vi "UHR-Fleezers Control (host) - 11.8.vi"() -> ()   [LabVIEW 2014] (continued)
  # "Rate param is ul/h\nVolume param is ul"
  # "Chemyx Pump 2"
  # "Units: \n1 = ml/m\n2 = ml/h\n3 = ul/m\n4 = ul/h"
  # "X"
  # "Y"
  # "Oscillate Set 1 freq. (debugging)"
  # "BD 1"
  # "BD 2"
  # "AOD Raster Scan"
  # "Approx. trap separations"
  # "X"
  # "Y"
  # "FPGA\nreading"
  # "DMA\ntransfer"
  # "APD Gates"
  # "APD 2"
  # "APD 1"
  # "X"
  # "2D"
  # "Y"
  # "1D"
  # "Green Laser Interlacing"
  # "Green FB Measurement"
  # "Digital Gate"
  # "Current Analog Control"
  # "Total AI Rates (NOT rates/trap)"
  # "(Samples/trap x Trap Sets)"
  # "(Samples/channel x\n8 if averaging (8 channels)\n4 if no averaging)"
  # "Trap 1"
  # "Trap 2"
  # "Flour./Trap 3"
  # "External Video Window"
  # "MCL Position Debugging"
  # "Temporary Control Storage\n(these used to be somewhere else, still want to keep them)"
  # "Y"
  # "X"
  # "Trap Position Difference Limits"
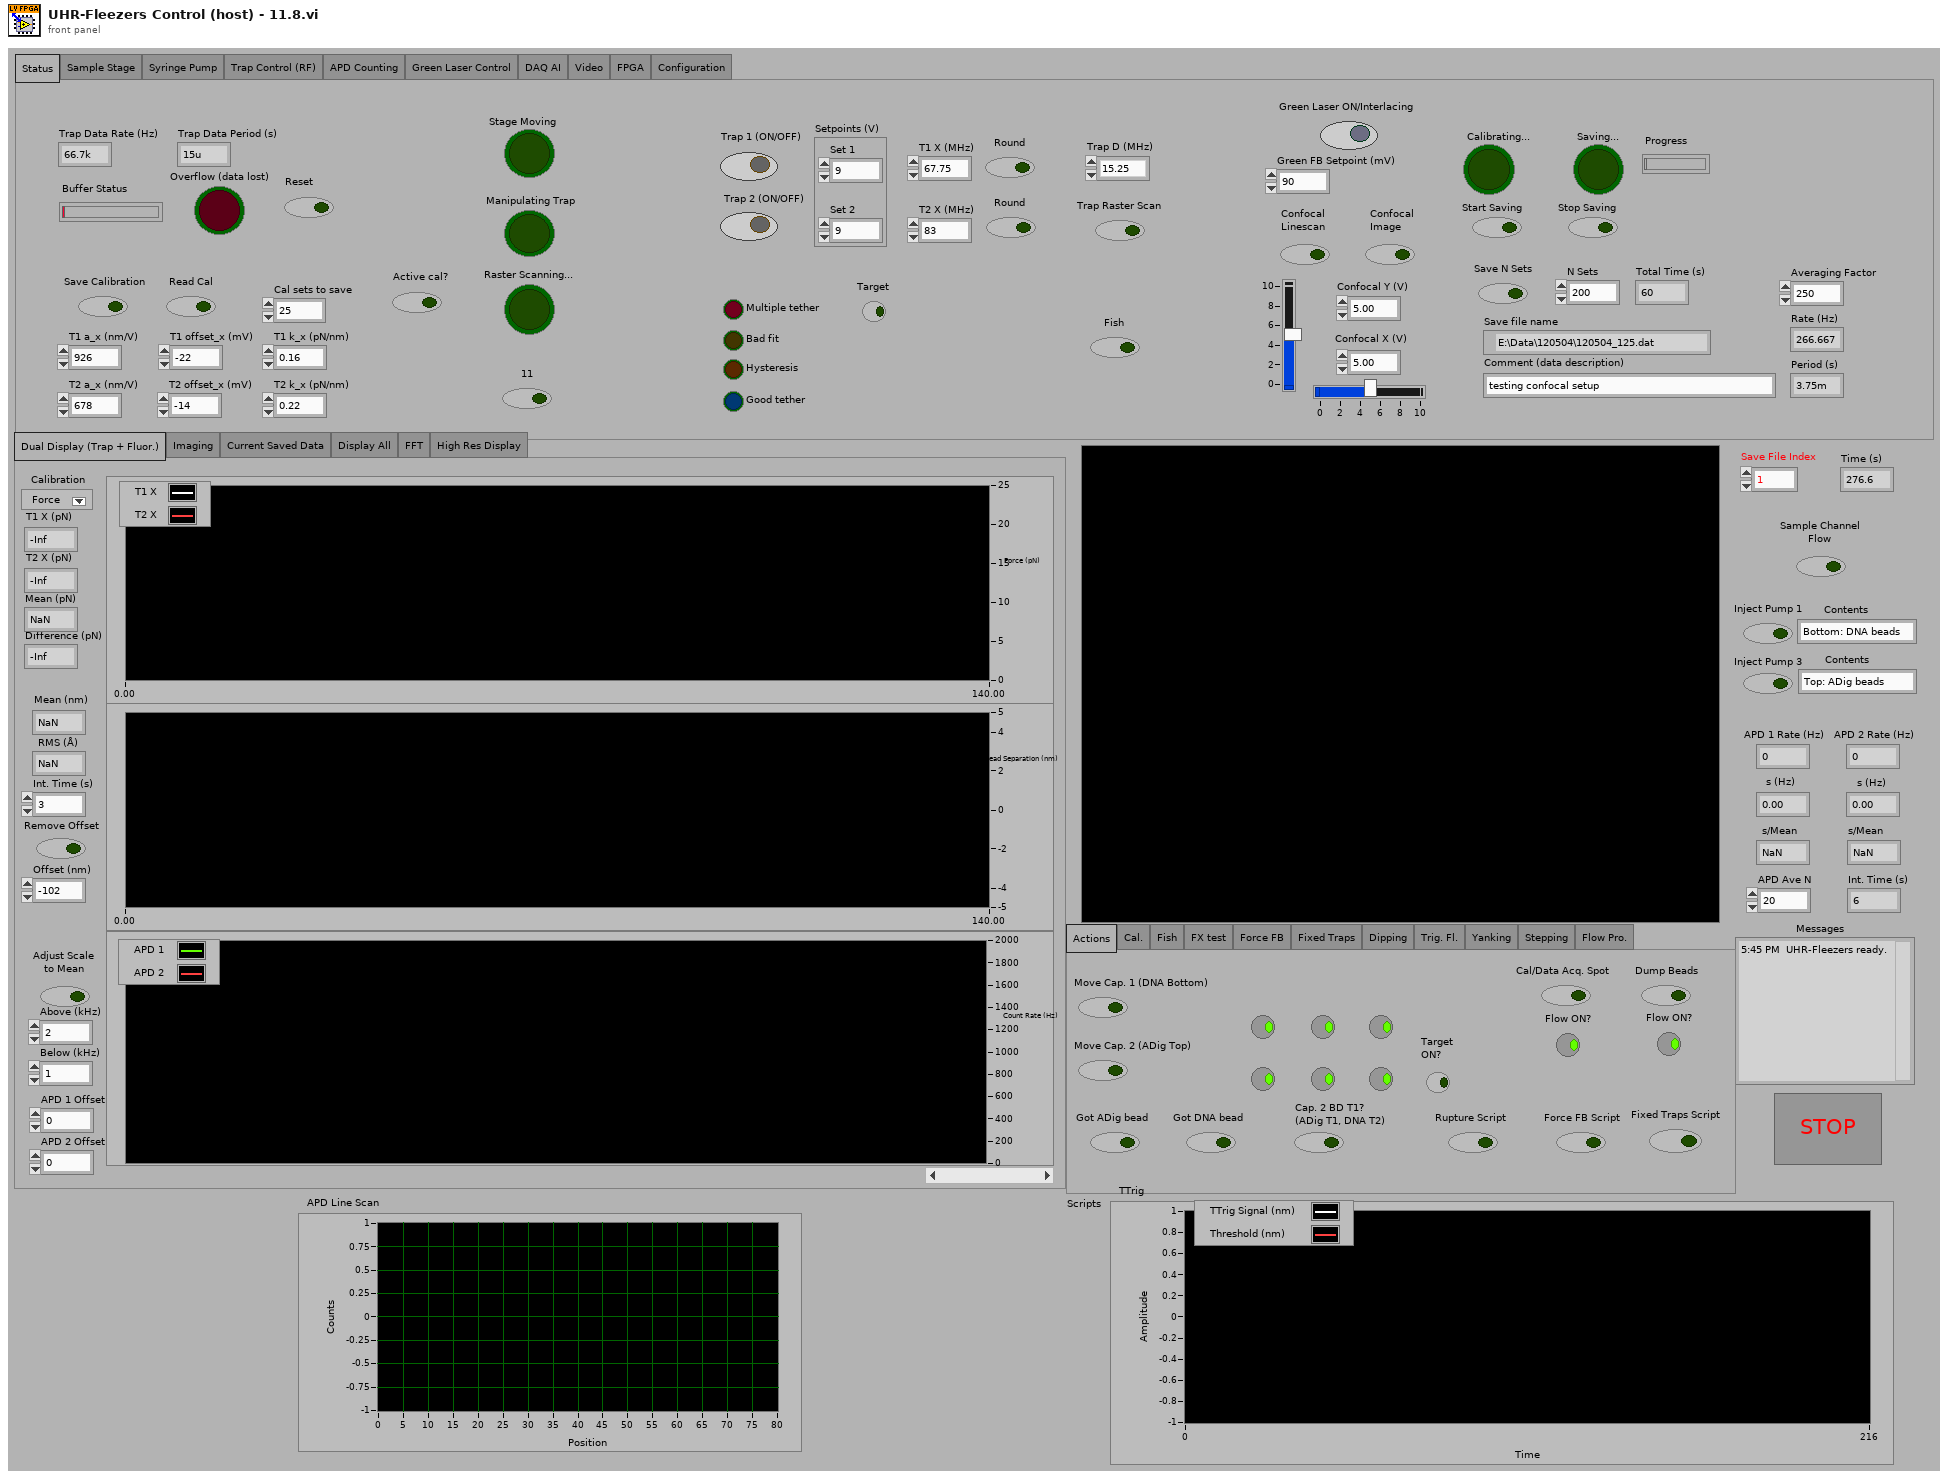
[diagram p1: front panel]
types:
  T1 = enum32{"Actions", "Cal.", "Fish", "FX test", "Force FB", "Fixed Traps", "Dipping", "Trig. Fl.", "Yanking", "Stepping", "Flow Pro."}
  T2 = typedef "IMAQ Image.ctl" = refnum<image>
  T3 = enum32{"Dual Display (Trap + Fluor.)", "Imaging", "Current Saved Data", "Display All", "FFT", "High Res Display"}
  T4 = enum32{"Status", "Sample Stage", "Syringe Pump", "Trap Control (RF)", "APD Counting", "Green Laser Control", "DAQ AI", "Video", "FPGA", "Configuration"}
  T5 = cluster{"Pump 1":cluster{"Diameter (mm)":dbl, "Units":dbl, "Volume":dbl, "Rate":dbl}, "Pump 2":cluster{"Diameter (mm)":dbl, "Units":dbl, "Volume":dbl, "Rate":dbl}, "Pump 3":cluster{"Diameter (mm)":dbl, "Units":dbl, "Volume":dbl, "Rate":dbl}}
  T6 = enum32{"IR Laser Interlacing (Direct RF Board Control Method)", "AOD Raster Scan", "Feedback on Trap Intensity", "Feedback on Trap Position"}
  T7 = typedef "LVPoint32TypeDef.ctl" = cluster{"Horizontal":i32, "Vertical":i32}
  T8 = cluster{"Scan Range AOD (nm) 2":dbl, "Step Size AOD (nm) 2":dbl, "Scan Speed AOD (nm/s) 2":dbl, "Number of scans (AOD) 2":u16, "Label":string}[]
  T9 = cluster{"Set 1":cluster{"proportional gain (Kc)":i16, "integral gain (Kc*Ts/Ti)":i16, "derivative gain (Kc*Td/Ts)":i16}, "Set 2":cluster{"proportional gain (Kc)":i16, "integral gain (Kc*Ts/Ti)":i16, "derivative gain (Kc*Td/Ts)":i16}}
  T10 = cluster{"Trap 1":fxp<+/-,16,1>, "Trap 2":fxp<+/-,16,1>}
  T11 = cluster{"proportional gain (Kc)":fxp<+/-,16,8>, "integral gain (Kc*Ts/Ti)":fxp<+/-,16,8>, "derivative gain (Kc*Td/Ts)":fxp<+/-,16,8>}
  T12 = cluster{"output high":fxp<+/-,64,32>, "output low":fxp<+/-,64,32>}
  T13 = cluster{"Set 1":fxp<+/-,16,1>, "Set 2":fxp<+/-,16,1>}
  T14 = cluster{"proportional gain (Kc)":i16, "integral gain (Kc*Ts/Ti)":i16, "derivative gain (Kc*Td/Ts)":i16}
  T15 = cluster{"Set 1":bool, "Set 2":bool, "Set 3":bool}
  T16 = typedef "LVMinMaxIncTypeDef.ctl" = cluster{"Minimum":dbl, "Maximum":dbl, "Increment":dbl}
  T17 = typedef "Image Type" = u32
  T18 = typedef "nirio_resource_hc.ctl" = tag
  T19 = typedef "openfpgaref.8.6.ctl" = refnum<k20>
  T20 = cluster{"New Image":T2, "New Image":T2, "New Image":T2, "New Image":T2}
  T21 = typedef "XDNodeRunTimeDep.lvlib/timing_clust.ctl" = cluster{"Expected End [f-1]":u64, "Actual End [f-1]":u64, "Finished Late? [f-1]":bool, "Expected End [i-1]":u64, "Actual End [i-1]":u64, "Finished Late? [i-1]":bool, "Expected Start [i]":u64, "Actual Start [i]":u64, "Expected Start [f]":u64, "Actual Start [f]":u64, "Source Name":string, "Structure Name":string, "Period":i64, "Deadline":i64, "Offset":i64, "Start":i64, "Priority":i32, "Timeout":i32, "Mode":T22, "Wakeup Reason":T23, "Error":errorcluster, "Source Type":string, "Secondary Source Type":string, "Global End Time":u64, "Global Start Time":u64, "Frame Duration":u64, "Iteration Duration":u64, "Assigned CPU":i32, "I/O Scan Engine Mode":u32}
  T22 = typedef "XDNodeRunTimeDep.lvlib/nitl_modes.ctl" = enum32{"No Change", "Process missed periods, maintain original phase", "Discard missed periods, maintain original phase", "Process missed periods, ignore original phase", "Discard missed periods, ignore original phase"}
  T23 = typedef "XDNodeRunTimeDep.lvlib/wakeup.ctl" = enum32{"Normal", "Aborted", "Asynchronous wakeup", "Timing source error", "Timed loop error", "Timeout"}
  T24 = enum16{"big-endian, network order", "native, host order", "little-endian"}
  T25 = enum16{"open", "replace", "create", "open or create", "replace or create", "replace or create with confirmation"}
  T26 = cluster{"Scan Range AOD (nm) 2":dbl, "Step Size AOD (nm) 2":dbl, "Scan Speed AOD (nm/s) 2":dbl, "Number of scans (AOD) 2":u16, "Label":string}
  T27 = cluster{"[0]":dbl, "[1]":dbl, "[2]":dbl, "[3]":dbl, "[4]":dbl, "[5]":dbl}
  T28 = cluster{"Diameter (mm)":dbl, "Units":dbl, "Volume":dbl, "Rate":dbl}
  T29 = enum16{"Actions", "Cal.", "Fish", "FX test", "Force FB", "Fixed Traps", "Dipping", "Trig. Fl.", "Yanking", "Stepping", "Flow Pro."}
  T30 = cluster{"Left":i32, "Top":i32, "Width":u32, "Height":u32}
  T31 = cluster{cluster{"Left":i32, "Top":i32, "Width":u32, "Height":u32}}[]
  T32 = enum32{"setting", "request", "request control", "info", "statistics", "system settings", "I/O sub system", "HRT control", "camera descriptions", "device specific data", "event sub system settings", "event sub system results", "image memory manager"}
  T33 = typedef "AviRefnum.ctl" = refnum<k1>
  T34 = typedef "imagedata.ctl" = cluster{"image type":i32, "image depth":i32, "image":u8[], "mask":u8[], "colors":u32[], "Rectangle":cluster{"left":i16, "top":i16, "right":i16, "bottom":i16}}
  T35 = enum32{"Normal Display", "Dual Display (APD)", "FFT", "High Res Display"}
  T36 = cluster{"Origin Pixel":cluster{"X":sgl, "Y":sgl}, "Angle Relative to Horizontal (deg)":sgl, "Axis Reference":u32}
  T37 = typedef "Simple Grid Descriptor" = cluster{"X Step":sgl, "Y Step":sgl, "Unit":T38}
  T38 = typedef "Image Unit" = enum32{"Undefined", "Angström", "Micrometer", "Millimeter", "Centimeter", "Meter", "Kilometer", "Microinch", "Inch", "Feet", "Nautical miles", "Standard miles", "Steps"}
  T39 = cluster{"averaging mode":u16, "weighting mode":u16, "number of averages":u32}
  T40 = cluster{"dB On (F)":bool, "unwrap phase (F)":bool, "convert to degree (F)":bool}
  T41 = cluster{string, string, string, string, string, string, string, string}
  T42 = cluster{string, string, string, string, string, string, string, string, string, string, string, string}
  T43 = cluster{string, string, string, string, string, string, string, string, string, string, string, string, string}
  T44 = cluster{string, string, string, string, string, string, string, string, string, string, string, string, string, string}
  T45 = cluster{"BD 1 Frequency 1 (MHz)":dbl, "BD 1 Frequency 2 (MHz)":dbl}
  T46 = cluster{"f0":dbl, "df":dbl, "magnitude":dbl[]}[][]
  T47 = cluster{"Green FB Ch 0":i16, "Green FB Ch 1":i16, "Green FB Ch 2":i16}
  T48 = cluster{"Green FB Ch 0":dbl, "Green FB Ch 1":dbl, "Green FB Ch 2":dbl}
diagram:
  w12 = 0.0 ("Total Volume\nFlowed P1 (uL)")
  w24 = u16 20 items=["1.0"=10, "1.5"=15, "2.0"=20] ("stop bits (10: 1 bit)")
  w27 = u16 20 items=["1.0"=10, "1.5"=15, "2.0"=20] ("stop bits (10: 1 bit)")
  w84 = u16 20 items=["1.0"=10, "1.5"=15, "2.0"=20] ("stop bits (10: 1 bit)")
  w91 = T17 2 items=["Grayscale (U8)", "Grayscale (I16)", "Grayscale (SGL)", "Complex (CSG)", "RGB (U32)", "HSL (U32)", "RGB (U64)", "Grayscale (U16)"] ("Image Type")
  w153 = cluster{"output high":i16, "output low":i16} {"output high"=3000, "output low"=0} ("FB output range 1")
  w224 = 10.0 ("y")
  w223 = 32767.0 ("y")
  w239 = 6.0  # clock mult.
  w240 = 49152000.0  # TCXO frequ.
  # "Bottom 1 Harvard"
  # "Top 3 Harvard"
  # "Center Harvard"
  # "Bottom 1 Harvard"
  # "Top 3 Harvard"
  # "Center Harvard"
  n1 = Build Array("DIO count 1 (ticks)", "DIO count 2 (ticks)", "DIO count 3 (ticks)") -> (w140:u32[])
  n2 = local read "AO1"() -> (w218:dbl)
  n3 = local read "AO2"() -> (w217:dbl)
  n4 = local read "Scan Increment (MHz)"() -> (w235:dbl)
  n5 = local read "Continuous MCL Scanning"() -> (w205:bool)
  n6 = local read "Fast Scan Dir"() -> (w204:bool)
  n7 = local read "Number of scans (MCL)"() -> (w206:u64)
  n8 = property on="AI Count (ticks)" class="DigNum (strict)"("Val(Sgnl)"="AI Count (ticks)") -> ()  [unwired: 2 in, 2 out]
  n9 = Multiply(x=w218, y=w223) -> (x*y=w220:dbl)
  n10 = Multiply(x=w217, y=w223) -> (x*y=w222:dbl)
  n11 = Divide(x=w220, y=w224) -> (x/y=w219:dbl)
  n12 = Divide(x=w222, y=w224) -> (x/y=w221:dbl)
  n13 = To Word Integer(number=w219) -> (16bit integer=w216:i16)
  n14 = To Word Integer(number=w221) -> (16bit integer=w215:i16)
  n15 = Not(x=w204) -> (.not. x?=w199:bool)
  n16 = local read "Cycles/step (MCL)"() -> (w207:u64)
  n17 = Multiply(x=w235, y=1000.0) -> (x*y=w242:dbl)
  n18 = local read "Scan steps (MCL)"() -> (w208:u64)
  n19 = local write "Trap Pos FIFO Timeout"(u16 0 ("Trap Pos FIFO Timeout")) -> ()
  n20 = local read "Desired Scan Incr (V)"() -> (w210:dbl)
  n21 = Scale By Power Of 2(n=48, x=w242) -> (x*2^n=w243:dbl)
  n22 = Multiply(x=w240, y=w239) -> (x*y=w238:dbl)
  n23 = Divide(x=w243, y=w238) -> (x/y=w237:dbl)
  n24 = local read "Setpoints (V)"() -> (w254:cluster{"Set 1":dbl, "Set 2":dbl})
  n25 = To Quad Integer(1:w237) -> (0:w234:i64)
  n26 = Divide(x=40000000.0, y="AI Count (ticks)") -> (x/y=w195:dbl)
  n27 = Multiply(x=w210, y=32767.0) -> (x*y=w212:dbl)
  n28 = local read "Number Interlace Sets"() -> (w133:u8)
  n29 = Split 1D Array(array=w140, index=w133) -> (first subarray=w142:u32[])  [unwired: 1 out]
  n30 = Add Array Elements(numeric array=w142) -> (sum=w141:u32)
  n31 = local read "# Samples/channel"() -> (w227:u32)
  n32 = local read "Number of F/B Scans (AOD)"() -> (w228:u16)
  n33 = local read "Not-Interlacing Set"() -> (w132:enum32{"Set 1", "Set 2", "Set 3"})
  n34 = To Unsigned Byte Integer(number=w132) -> (unsigned 8bit integer=w138:u8)
  n35 = Index Array(array=w140, index=w138) -> (element=w139:u32)
  n36 = local read "Feedback On/Off"() -> (w257:cluster{"Set 1":bool, "Set 2":bool})
  n37 = local read "PID Gains"() -> (w249:T9)
  n38 = local read "Scan steps (AOD)"() -> (w233:u64)
  n39 = local read "All FB On/Off"() -> (w258:bool)
  n40 = local read "Cycles/step (AOD)"() -> (w232:u64)
  n41 = local write "AI rate (Hz)"(w195) -> ()
  n42 = Divide(x=w212, y=10.0) -> (x/y=w211:dbl)
  n43 = Multiply(x=w233, y=w232) -> (x*y=w231:u64)
  n44 = Multiply(x=3276.7, y=w254) -> (x*y=w253:cluster{"Set 1":dbl, "Set 2":dbl})
  n45 = To Word Integer(number=w211) -> (16bit integer=w209:i16)
  n46 = xnode "Open FPGA VI Reference"("resource name"=T18 "RIO1") -> ("FPGA VI Reference Out"=w10:T19, "error out"=w8:errorcluster)  [unwired: 1 in]
  n47 = Multiply(x=w231, y=u64 2) -> (x*y=w229:u64)
  n48 = local read "Sets to FIFO (Traps)"() -> (w261:T15)
  n49 = Divide(x=w195, y="FPGA Ave.") -> (x/y=w196:dbl)
  n50 = To Word Integer(number=w253) -> (16bit integer=w252:cluster{"Set 1":i16, "Set 2":i16})
  n51 = Unbundle By Name(w249) -> ("Set 1"=w248:T14, "Set 2"=w247:T14)
  n52 = Multiply(x=w229, y=w228) -> (x*y=w226:u64)
  n53 = local write "Ave. Rate (Hz)"(w196) -> ()
  n54 = Divide(x=w226, y=w227) -> (x/y=w225:dbl)
  n55 = Unbundle By Name(w252) -> ("Set 1"=w251:i16, "Set 2"=w250:i16)
  n56 = local read "2D or 1D Scan"() -> (w154:bool)
  n57 = local write "Data points/scans"(w226) -> ()
  n58 = local read "Scan BD"() -> (w244:bool)
  n59 = And(x=w257, y=w258) -> (x .and. y?=w256:cluster{"Set 1":bool, "Set 2":bool})
  n60 = local write "Data points/scan (f/b)"(w229) -> ()
  n61 = Reciprocal(x=w196) -> (1/x=w197:dbl)
  n62 = local read "N Acq Sets (Traps + Fl.)"() -> (w188:i16)
  n63 = local write "N sets should be saved"(w225) -> ()
  n64 = xnode "Invoke Method"("FPGA VI Reference In"=w10, "error in"=w8) -> ("FPGA VI Reference Out"=w152:T19, "error out"=w162:errorcluster)
  n65 = Unbundle By Name(w256) -> ("Set 1"=w260:bool, "Set 2"=w259:bool)
  n66 = local read "Interlace"() -> (w134:bool)
  n67 = Select(t=w141, s=w134, f=w139) -> (s? t:f=w131:u32)
  n68 = local write "Update Count (MCL)"(w131) -> ()
  n69 = local write "Total Counts (ticks)"(w131) -> ()
  n70 = local write "Ave. Period (s)"(w197) -> ()
  n71 = property on="2D or 1D Scan" class="Bool (strict)"("Val(Sgnl)"=w154) -> ()  [unwired: 2 in, 2 out]
  n72 = local read "GI Frequency, OFF count"() -> (w56:u32)
  n73 = local read "GI Frequency, ON count"() -> (w47:u32)
  n74 = local read "APD Gate OFF Count"() -> (w53:u32)
  n75 = local read "APD Gate ON Count"() -> (w49:u32)
  n76 = xnode "Read/Write Control"("FPGA VI Reference In"=w151, "error in"=w162, "ai count"="AI Count (ticks)", "Interlace ON/OFF"=w134, "Number Interlace Cycles"=w133, "AI1 Sets to FIFO"=w261, "FB On/Off Set 1"=w260, "FB On/Off Set 2"=w259, "Interlace Off Parameters"=w132, "FB Setpoint Set 1"=w251, "FB Setpoint Set 2"=w250, "FB Gains Set 1"=w248, "FB Gains Set 2"=w247, "FB output range 1"=w153, "FB output range 2"=w153, "Cycles per step"=w232, "Scan BD"=w244, "Number of scans"=w228, "Scan steps"=w233, "Scan freq.  increment"=w234, "AO1"=w216, "AO2"=w215, "Scan freq.  increment (MCL)"=w209, "Scan steps (MCL)"=w208, "Cycles per step (MCL)"=w207, "Number of scans (MCL)"=w206, "MCL count"=w131, "Cont. Scan (MCL)"=w205, "MCL Scan Axis"=w199, "1D or 2D Scan?"=w154, "N of AI1 Int Acq Sets"=w188, "Freq or Amp switch first"="Freq or Amp switch first", "Freq switch delay"="Freq switch delay", "Amp switch delay"="Amp switch delay", "Swap F1 and F2"="Swap F1 and F2", "APD to FIFO"=FALSE, "DIO count 1 (ticks)"="DIO count 1 (ticks)", "DIO count 2 (ticks)"="DIO count 2 (ticks)", "DIO count 3 (ticks)"="DIO count 3 (ticks)") -> ("FPGA VI Reference Out"=w60:T19, "error out"=w58:errorcluster)  [unwired: 1 in]
  n77 = local read "On one out of X cycles"() -> (w55:u32)
  n78 = local read "APD Integration Time (s)"() -> (w39:dbl)
  n79 = local read "DMA Update Period (s)"() -> (w38:dbl)
  n80 = Add(x=w49, y=w53) -> (x+y=w51:u32)
  n81 = Add(x=w47, y=w56) -> (x+y=w54:u32)
  n82 = local read "Green Laser ON/Interlacing"() -> (w129:bool)
  n83 = local read "Green laser mode"() -> (w130:enum32{"Laser ON", "Laser OFF", "Interlace"})
  n84 = Multiply(x=w51, y=w55) -> (x*y=w52:u32)
  n85 = Multiply(x=w55, y=w54) -> (x*y=w46:u32)
  n86 = Reciprocal(x=w39) -> (1/x=w36:dbl)
  n87 = Multiply(x=w39, y=40000000.0) -> (x*y=w35:dbl)
  n88 = Divide(x=w38, y=w39) -> (x/y=w41:dbl)
  n89 = Multiply(x="Current When FB OFF (%)", y=655.35) -> (x*y=w117:dbl)
  n90 = local read "Invert APD Gate"() -> (w45:bool)
  n91 = Multiply(x="Green FB Setpoint (mV)", y=3.2767) -> (x*y=w114:dbl)
  n92 = local read "APD Gate"() -> (w44:enum32{"ON", "OFF", "Interlace"})
  n93 = Subtract(x=w52, y=w49) -> (x-y=w50:u32)
  n94 = local write "Green FB Count"(w46) -> ()
  n95 = local write "APD Acq Rate (Hz)"(w36) -> ()
  n96 = To Unsigned Long Integer(number=w35) -> (unsigned 32bit integer=w33:u32)
  n97 = Multiply(x=2.0, y=w41) -> (x*y=w40:dbl)
  n98 = local read "Invert GI"() -> (w126:bool)
  n99 = To Unsigned Word Integer(number=w117) -> (unsigned 16bit integer=w115:u16)
  n100 = Subtract(x=w46, y=w47) -> (x-y=w48:u32)
  n101 = local write "APD Samples/FIFO Acq."(w41) -> ()
  n102 = To Word Integer(number=w114) -> (16bit integer=w112:i16)
  n103 = local write "APD Elements/DMA read"(w40) -> ()
  n104 = case shown="False" w129 {
    tunnel: w130 -> [_ w286]
    tunnel: [enum32{"Laser ON", "Laser OFF", "Interlace"}."Laser OFF" ("Green laser mode") w286] -> w125
    frame False {
    }
    frame True {
    }
  }
  n105 = local write "APD Int. Count"(w33) -> ()
  n106 = local read "Trap Pos. AI1 X Pre-scale"() -> (w70:u16)
  n107 = local read "Trap Pos FB Monitor\nT1 or T2"() -> (w77:bool)
  n108 = local read "Trap Pos FB Int Count"() -> (w64:u16)
  n109 = local read "APD 1 AO Mult."() -> (w43:i16)
  n110 = local read "Trap Pos FB Negate Action"() -> (w76:bool)
  n111 = local read "APD 2 AO Mult."() -> (w42:i16)
  n112 = local read "Trap Pos. FB Offset Factor"() -> (w75:i64)
  n113 = local read "Trap Pos. FB Mult Factor"() -> (w74:i64)
  n114 = local read "Differential FB?"() -> (w30:bool)
  n115 = local read "Neg. TTrig FPGA"() -> (w32:bool)
  n116 = local read "Trap Pos. FB Gains"() -> (w72:T11)
  n117 = local read "Trap Pos. FB Range"() -> (w73:T12)
  n118 = xnode "Read/Write Control"("FPGA VI Reference In"=w60, "error in"=w58, "Invert APD Gate"=w45, "APD Gate ON Count"=w49, "APD Gate OFF Count"=w50, "APD Acq Rate Count"=w33, "APD Gate Operating Mode"=w44, "APD 1 AO scale factor"=w43, "APD 2 AO scale factor"=w42, "Green interlace ON count"=w47, "Green interlace OFF count"=w48, "Green interlace ON count 2"=w47, "Green interlace OFF count 2"=w48, "Green FB Count"=w46) -> ("FPGA VI Reference Out"=w59:T19, "error out"=w57:errorcluster)
  n119 = xnode "Read/Write Control"("FPGA VI Reference In"=w59, "error in"=w57, "Invert GI 2"=w126, "Operating Mode 2"=w125, "Green FB Gains"="Green FB Gains", "Green FB Setpoint"=w112, "Green FB On/Off"="Green FB On/Off", "Current Out"=w115, "Green int current ON count adj"="Green int current ON count adj", "Operating Mode"=w125, "Invert GI"=w126, "Trap Pos FB Monitor T1 or T2"=w77, "Trap Pos FB Negate Action"=w76, "Trap Pos. FB Offset Factor"=w75, "Trap Pos. FB Mult Factor"=w74, "Trap Pos. FB Range"=w73, "Trap Pos. FB Gains"=w72, "Force feedback"=FALSE, "AI1 X Scale"=w70, "Trap Pos to FIFO"=TRUE, "Trap Pos FB Int Count"=w64, "TTrig Negate Pos"=w32, "FB Trig Integrate"="FB Trig Integrate", "Diff FB Measurement?"=w30, "Negate Diff?"="Negate Diff?") -> ("FPGA VI Reference Out"=w127:T19, "error out"=w128:errorcluster)
  n120 = xnode "Invoke Method"("FPGA VI Reference In"=w127, "error in"=w128, "Requested Depth"="Trap AI FIFO Depth") -> ("FPGA VI Reference Out"=w80:T19, "error out"=w79:errorcluster)  [unwired: 1 out]
  n121 = xnode "Invoke Method"("FPGA VI Reference In"=w80, "error in"=w79, "Requested Depth"="Trap Position FIFO Depth") -> ("FPGA VI Reference Out"=w66:T19, "error out"=w65:errorcluster)  [unwired: 1 out]
  n122 = flat-sequence {
    tunnel: w152 -> [w291]
    tunnel: [w291] -> w151
    tunnel: [w290] -> w150
    tunnel: [w289] -> w149
    tunnel: [w287] -> w147
    tunnel: [w288] -> w148
    frame #0 {
      w288 = T16 {"Minimum"=0.0, "Maximum"=40.0, "Increment"=1.0} ("Min Max Inc")
      w287 = T16 {"Minimum"=0.0, "Maximum"=50.0, "Increment"=1.0} ("Data Entry Limits")
      w290 = T16 {"Minimum"=60.0, "Maximum"=90.0, "Increment"=1.0} ("Min Max Inc")
      w289 = T16 {"Minimum"=0.0, "Maximum"=50.0, "Increment"=1.0} ("Data Entry Limits")
      n123 = property on="BD 2 Frequency 1 (MHz)" class="DigNum (strict)"("Data Range"=w288) -> ()  [unwired: 2 in, 2 out]
      n124 = property on="BD 2 Frequency 3 (MHz)" class="DigNum (strict)"("Data Range"=w288) -> ()  [unwired: 2 in, 2 out]
      n125 = property on="BD 2 Frequency 2 (MHz)" class="DigNum (strict)"("Data Range"=w288) -> ()  [unwired: 2 in, 2 out]
      n126 = property on="BD 1 Frequency 1 (MHz)" class="DigNum (strict)"("Data Range"=w290) -> ()  [unwired: 2 in, 2 out]
      n127 = property on="BD 1 Frequency 2 (MHz)" class="DigNum (strict)"("Data Range"=w290) -> ()  [unwired: 2 in, 2 out]
      n128 = property on="BD 1 Frequency 3 (MHz)" class="DigNum (strict)"("Data Range"=w290) -> ()  [unwired: 2 in, 2 out]
      n129 = property on="BD 2 Amplitude 1 (%)" class="DigNum (strict)"("Data Range"=w287) -> ()  [unwired: 2 in, 2 out]
      n130 = property on="BD 2 Amplitude 2 (%)" class="DigNum (strict)"("Data Range"=w287) -> ()  [unwired: 2 in, 2 out]
      n131 = property on="BD 2 Amplitude 3 (%)" class="DigNum (strict)"("Data Range"=w287) -> ()  [unwired: 2 in, 2 out]
      n132 = property on="BD 1 Amplitude 3 (%)" class="DigNum (strict)"("Data Range"=w289) -> ()  [unwired: 2 in, 2 out]
      n133 = property on="BD 1 Amplitude 2 (%)" class="DigNum (strict)"("Data Range"=w289) -> ()  [unwired: 2 in, 2 out]
      n134 = property on="BD 1 Amplitude 1 (%)" class="DigNum (strict)"("Data Range"=w289) -> ()  [unwired: 2 in, 2 out]
      "X RF Frequency Limits (MHz)" <- w290
      "X RF Amplitude Limits (%)" <- w289
      "Y RF Amplitude Limits (%)" <- w287
      "Y RF Frequency Limits (MHz)" <- w288
    }
  }
  n135 = xnode "Invoke Method"("FPGA VI Reference In"=w66, "error in"=w65) -> ("FPGA VI Reference Out"=w161:T19, "error out"=w160:errorcluster)  [unwired: 1 in]
  n136 = flat-sequence "Initial FPGA Loop Relative Phase Adjustment" {
    tunnel: "Initial Phase Adjustment (APD 2 Gate)" -> [w294]
    tunnel: "Initial Phase Adjustment (GI) 2" -> [w295]
    tunnel: "Initial Phase Adj. (MCL)" -> [w293]
    tunnel: w160 -> [w296]
    tunnel: w161 -> [w297]
    tunnel: "Initial Phase Adjustment (GI)" -> [w298]
    tunnel: "Initial Phase Adjustment (AI1)" -> [w299]
    tunnel: [w299] -> w7
    tunnel: [w298] -> w6
    tunnel: [w297] -> w5
    tunnel: [w296] -> w4
    tunnel: [w293] -> w3
    tunnel: [w295] -> w2
    tunnel: [w294] -> w1
    tunnel: [w311] -> w170
    tunnel: [w305] -> w166
    tunnel: "Initial Phase Adjustment (APD Acq)" -> [w304]
    tunnel: "Initial Phase Adjustment (APD 1 Gate)" -> [w303]
    tunnel: "Initial Phase Adjustment (Green FB)" -> [w302]
    tunnel: w7 -> [w310]
    tunnel: w6 -> [w309]
    tunnel: w5 -> [w308]
    tunnel: w4 -> [w307]
    tunnel: w3 -> [w306]
    tunnel: w2 -> [w301]
    tunnel: w1 -> [w300]
    tunnel: w170 -> [w313]
    tunnel: [w314] -> w167
    tunnel: w166 -> [w314]
    tunnel: [w313] -> w165
    tunnel: w167 -> [w317]
    tunnel: w165 -> [w316]
    tunnel: [w319] -> w164
    tunnel: [w318] -> w163
    tunnel: [w321] -> w168
    tunnel: [w322] -> w169
    tunnel: w164 -> [w322]
    tunnel: w163 -> [w321]
    frame #0 {
      n137 = Wait (ms)(milliseconds to wait=u32 100) -> ()  [unwired: 1 out]
    }
    frame #1 {
      n138 = xnode "Read/Write Control"("FPGA VI Reference In"=w308, "error in"=w307, "Phase count adjustment"=w310, "Phase count adjustment (GI)"=w309, "Phase count adjustment (MCL)"=w306, "Phase Count Adjustment (APD Acq)"=w304, "Phase count adjustment (APD 1 Gate)"=w303, "Phase count adjustment (APD 2 Gate)"=w300, "Phase count adjustment (Green FB)"=w302, "Phase count adjustment (GI) 2"=w301) -> ("FPGA VI Reference Out"=w305:T19, "error out"=w311:errorcluster)
    }
    frame #2 {
      n139 = Wait (ms)(milliseconds to wait=u32 100) -> ()  [unwired: 1 out]
    }
    frame #3 {
      w315 = TRUE
      n140 = xnode "Read/Write Control"("FPGA VI Reference In"=w317, "error in"=w316, "+ phase"=w315, "+ phase (GI)"=w315, "+ phase (MCL)"=w315, "+ phase (APD Acq)"=w315, "+ phase (APD 1 Gate)"=w315, "+ phase (APD 2 Gate)"=w315, "+ phase (Green FB)"=w315, "+ phase (GI) 2"=w315) -> ("FPGA VI Reference Out"=w318:T19, "error out"=w319:errorcluster)
    }
    frame #4 {
      n141 = Wait (ms)(milliseconds to wait=u32 100) -> ()  [unwired: 1 out]
    }
  }
  n142 = local read "Phase adj. (Green FB)"() -> (w143:i16)
  n143 = local read "Phase adj. (GI) 2"() -> (w118:i16)
  n144 = local read "Phase adjust (MCL)"() -> (w200:i16)
  n145 = local read "Phase adj. (AI1)"() -> (w202:i16)
  n146 = local read "Phase adj. (GI)"() -> (w201:i16)
  n147 = xnode "Read/Write Control"("FPGA VI Reference In"=w168, "error in"=w169, "Phase count adjustment"=w202, "Phase count adjustment (GI)"=w201, "Phase count adjustment (MCL)"=w200, "Phase Count Adjustment (APD Acq)"="Phase Adj. (APD Acq)", "Phase count adjustment (APD 1 Gate)"="Phase Adj. (APD 1 Gate)", "Phase count adjustment (APD 2 Gate)"="Phase Adj. (APD 2 Gate)", "Phase count adjustment (Green FB)"=w143, "Phase count adjustment (GI) 2"=w118) -> ("FPGA VI Reference Out"=w9:T19, "error out"=w177:errorcluster)
  n148 = call "Initialize RF boards - interlace 3.vi"("error in"=w177, "FPGA VI Reference In"=w9) -> ("error out"=w175:errorcluster, "FPGA VI Reference Out"=w176:T19)
  n149 = call "set RF board frequency - interlace.vi"("Board 2 Frequency Limits"=w148, "Board 1 Frequency Limits"=w150, "error in"=w175, "FPGA VI Reference In"=w176, "Board 2 Frequency 3 (MHz)"="BD 2 Frequency 3 (MHz)", "Board 1 Frequency 3 (MHz)"="BD 1 Frequency 3 (MHz)", "Board 2 Frequency 2 (MHz)"="BD 2 Frequency 2 (MHz)", "Board 2 Frequency 1 (MHz)"="BD 2 Frequency 1 (MHz)", "Board 1 Frequency 2 (MHz)"="BD 1 Frequency 2 (MHz)", "Board 1 Frequency 1  (MHz)"="BD 1 Frequency 1 (MHz)") -> ("error out"=w276:errorcluster, "FPGA VI Reference Out"=w277:T19)
  n150 = call "set RF board amplitude - interlace.vi"("Board 2 Amplitude Limits"=w147, "Board 1 Amplitude Limits"=w149, "error in"=w276, "FPGA VI Reference In"=w277, "Board 2 Amplitude 3 (%)"="BD 2 Amplitude 3 (%)", "Board 1 Amplitude 3 (%)"="BD 1 Amplitude 3 (%)", "Board 2 Amplitude 2 (%)"="BD 2 Amplitude 2 (%)", "Board 2 Amplitude 1 (%)"="BD 2 Amplitude 1 (%)", "Board 1 Amplitude 2 (%)"="BD 1 Amplitude 2 (%)", "Board 1 Amplitude 1 (%)"="BD 1 Amplitude 1 (%)") -> ("error out"=w264:errorcluster, "FPGA VI Reference Out"=w265:T19)
  n151 = flat-sequence {
    tunnel: w265 -> [w332]
    tunnel: w264 -> [w331]
    tunnel: [w330] -> w269
    tunnel: [w329] -> w268
    tunnel: [w336] -> w267
    tunnel: w269 -> [w336]
    tunnel: [w335] -> w266
    tunnel: w268 -> [w335]
    tunnel: w267 -> [w345]
    tunnel: w266 -> [w344]
    tunnel: [w343] -> w18
    tunnel: [w342] -> w67
    frame #0 {
      w323 = FALSE ("Retract Pump 3")
      n152 = local read "Trap 1 (ON/OFF)"() -> (w324:bool)
      n153 = xnode "Read/Write Control"("FPGA VI Reference In"=w332, "error in"=w331, "Direct RF Box  Communication"=FALSE) -> ("FPGA VI Reference Out"=w330:T19, "error out"=w329:errorcluster)
      n154 = local write "Saving..."(FALSE ("Saving Data")) -> ()
      n155 = local write "Stop All"(FALSE ("Stop All")) -> ()
      n156 = local write "Retract Pump 1"(w323) -> ()
      n157 = local write "Retract Pump 3"(w323) -> ()
      n158 = local write "Index"(1.0 ("Index")) -> ()
      n159 = property on="Trap 1 ON" class="Bool (strict)"("Value"=w324) -> ()  [unwired: 2 in, 2 out]
      "Manipulating Trap" <- FALSE ("Manipulating Trap")
    }
    frame #1 {
      n160 = local read "Trap 2 (ON/OFF)"() -> (w334:bool)
      n161 = Wait (ms)(milliseconds to wait=u32 10) -> ()  [unwired: 1 out]
      n162 = property on="Trap 2 ON" class="Bool (strict)"("Val(Sgnl)"=w334) -> ()  [unwired: 2 in, 2 out]
    }
    frame #2 {
      n163 = local read "Scan Range (nm)"() -> (w338:dbl)
      n164 = xnode "Read/Write Control"("FPGA VI Reference In"=w345, "error in"=w344, "FPGA Controls  RF Box"=TRUE ("Direct RF Box  Communication")) -> ("FPGA VI Reference Out"=w343:T19, "error out"=w342:errorcluster)
      n165 = call "Update messages.vi"("Message to add"="UHR-Fleezers ready.", "Old message string"="") -> ("New message string"=w341:string)
      n166 = local write "Messages"(w341) -> ()
      n167 = property on="Scan Range (nm)" class="DigNum (strict)"("Val(Sgnl)"=w338) -> ()  [unwired: 2 in, 2 out]
    }
  }
  n168 = Subtract(x="BD 1 Frequency 1 (MHz)", y="BD 1 Frequency 2 (MHz)") -> (x-y=w187:dbl)
  n169 = Subtract(x="BD 2 Frequency 1 (MHz)", y="BD 2 Frequency 2 (MHz)") -> (x-y=w186:dbl)
  n170 = Square(x=w186) -> (x^2=w184:dbl)
  n171 = Square(x=w187) -> (x^2=w185:dbl)
  n172 = Add(x=w185, y=w184) -> (x+y=w183:dbl)
  n173 = Square Root(x=w183) -> (sqrt(x)=w182:dbl)
  n174 = local write "Trap D (MHz)"(w182) -> ()
  n175 = call "IMAQ Create"("Image Name"="APD 1 Image", "Image Type"=w91) -> ("New Image"=w90:T2)  [unwired: 3 in, 1 out]
  n176 = call "IMAQ Create"("Image Name"="APD 2 Image", "Image Type"=w91) -> ("New Image"=w89:T2)  [unwired: 3 in, 1 out]
  n177 = call "IMAQ Create"("Image Name"="Det. X Image", "Image Type"=w91) -> ("New Image"=w88:T2)  [unwired: 3 in, 1 out]
  n178 = call "IMAQ Create"("Image Name"="Det. Y Image", "Image Type"=w91) -> ("New Image"=w87:T2)  [unwired: 3 in, 1 out]
  n179 = Bundle("New Image"=w90, "New Image"=w89, "New Image"=w88, "New Image"=w87) -> (w86:T20)  [unwired: 1 in]
  n180 = call-poly "VISA Configure Serial Port"("VISA resource name"="Bottom  1 Harvard Syringe Pump Serial Port", "baud rate (9600)"=u32 115200, "stop bits (10: 1 bit)"=w24) -> ("VISA resource name out"=w20:refnum<visa-resource-name>, "error out"=w19:errorcluster)  [unwired: 4 in, 7 out]
  n181 = call-poly "VISA Configure Serial Port"("VISA resource name"="Top 3 Harvard Syringe Pump Serial Port", "baud rate (9600)"=u32 115200, "stop bits (10: 1 bit)"=w27) -> ("VISA resource name out"=w22:refnum<visa-resource-name>, "error out"=w21:errorcluster)  [unwired: 4 in, 7 out]
  n182 = call-poly "VISA Configure Serial Port"("VISA resource name"="Sample Chamber Stage Serial Port") -> ("VISA resource name out"=w100:refnum<visa-resource-name>, "error out"=w101:errorcluster)  [unwired: 5 in, 8 out]
  "Stage Control Serial Error" <- w101
  n183 = call-poly "VISA Configure Serial Port"("VISA resource name"="Center Harvard Syringe Pump Serial Port", "baud rate (9600)"=u32 115200, "stop bits (10: 1 bit)"=w84) -> ("VISA resource name out"=w81:refnum<visa-resource-name>, "error out"=w82:errorcluster)  [unwired: 4 in, 7 out]
  n184 = disable-structure shown="Disabled" {
    disable-tunnel: [w348 _] -> w246
    disable-tunnel: w18 -> [w347 _]
    frame Disabled {
      n185 = node-c288() -> (w350:T21)  [unwired: 4 out]
      n186 = timed-loop "Rough control of MCL mirror stage (debugging)" {
        tunnel: w347 -> [w353]
        tunnel: [w352] -> w348
        timing: w350 -> [_]
        timing-out: [_] -> w349
        stop <- w352 stop-if-true
        n187 = node-c288() -> ()  [unwired: 2 out]
        n188 = case shown="1" "MCL Mode" {
          tunnel: w353 -> [_ w356 w403]
          frame 0, Default {
          }
          frame 1 {
            n189 = node-c288() -> (w358:T21)  [unwired: 4 out]
            n190 = timed-loop "Oscillate MCL mirror" {
              timing: w358 -> [_]
              timing-out: [_] -> w357
              tunnel: w356 -> [w397]
              i -> [w396]
              stop <- w359 stop-if-true
              n191 = node-c288() -> (w395:i64)  [unwired: 1 out]
              n192 = Multiply(x="AO1", y=32767.0) -> (x*y=w391:dbl)
              n193 = Multiply(x="AO2", y=32767.0) -> (x*y=w386:dbl)
              n194 = Divide(x=w391, y=10.0) -> (x/y=w392:dbl)
              n195 = Divide(x=w386, y=10.0) -> (x/y=w387:dbl)
              n196 = To Word Integer(number=w392) -> (16bit integer=w384:i16)
              n197 = To Word Integer(number=w387) -> (16bit integer=w383:i16)
              n198 = Divide(x=w395, y=i64 1000) -> (x/y=w366:dbl)
              n199 = Multiply(x=w366, y=w396) -> (x*y=w377:dbl)
              n200 = Multiply(x="Osc. freq. (Hz) 2", y=6.283185307179586) -> (x*y=w378:dbl)
              n201 = Multiply(x=w378, y=w377) -> (x*y=w376:dbl)
              n202 = Sine(x=w376) -> (sin(x)=w375:dbl)
              n203 = Multiply(x=w375, y="Osc. amp. (V)") -> (x*y=w373:dbl)
              n204 = Add(x=w373, y="Osc. center (V)") -> (x+y=w371:dbl)
              n205 = Divide(x=w371, y=10.0) -> (x/y=w369:dbl)
              n206 = Multiply(x=w369, y=32767.0) -> (x*y=w364:dbl)
              n207 = Select(t=w364, s="Scan axis", f=w384) -> (s? t:f=w382:dbl)
              n208 = Select(t=w383, s="Scan axis", f=w364) -> (s? t:f=w381:dbl)
              n209 = local read "MCL Mode"() -> (w363:u16)
              n210 = Not Equal?(x=w363, y=u16 1) -> (x != y?=w360:bool)
              n211 = local read "Stop All"() -> (w361:bool)
              n212 = xnode "Read/Write Control"("FPGA VI Reference In"=w397, "AO1"=w382, "AO2"=w381) -> ()  [unwired: 1 in, 2 out]
              n213 = Compound Arithmetic op=OR(w361, w360) -> (w359:bool)
              n214 = node-c288() -> ()  [unwired: 2 out]
            }
            n215 = node-c288(w357) -> ()  [unwired: 1 out]
          }
          frame 2 {
            n216 = case shown="True" "Start Scan" {
              tunnel: w403 -> [_ w415]
              frame False {
              }
              frame True {
                n217 = Subtract(x="End (V)", y="Begin (V)") -> (x-y=w411:dbl)
                n218 = Decrement(x="N Points") -> (x-1=w410:dbl)
                n219 = Divide(x=w411, y=w410) -> (x/y=w408:dbl)
                n220 = for {
                  N: "N Points" -> [_]
                  tunnel: "Begin (V)" -> [w428]
                  tunnel: w415 -> [w420]
                  tunnel: [w419] -> w414 mode=indexing
                  tunnel: w408 -> [w418]
                  tunnel: [w416] -> w407 mode=indexing
                  i -> [w427]
                  n221 = Multiply(x=w418, y=w427) -> (x*y=w426:dbl)
                  n222 = Add(x=w428, y=w426) -> (x+y=w423:dbl)
                  n223 = local read "Scan axis"() -> (w417:bool)
                  n224 = local read "AO1"() -> (w425:dbl)
                  n225 = local read "AO2"() -> (w424:dbl)
                  n226 = Select(t=w423, s=w417, f=w425) -> (s? t:f=w422:dbl)
                  n227 = Select(t=w424, s=w417, f=w423) -> (s? t:f=w421:dbl)
                  n228 = flat-sequence {
                    tunnel: w422 -> [w432]
                    tunnel: w421 -> [w431]
                    tunnel: w420 -> [w429]
                    tunnel: [w442] -> w419
                    tunnel: [w441] -> w416
                    frame #0 {
                      w435 = 10.0 ("y")
                      w430 = 32767.0 ("y")
                      n229 = Multiply(x=w432, y=w430) -> (x*y=w438:dbl)
                      n230 = Multiply(x=w431, y=w430) -> (x*y=w436:dbl)
                      n231 = Divide(x=w438, y=w435) -> (x/y=w439:dbl)
                      n232 = Divide(x=w436, y=w435) -> (x/y=w437:dbl)
                      n233 = To Word Integer(number=w439) -> (16bit integer=w433:i16)
                      n234 = To Word Integer(number=w437) -> (16bit integer=w434:i16)
                      n235 = xnode "Read/Write Control"("FPGA VI Reference In"=w429, "AO1"=w433, "AO2"=w434) -> ()  [unwired: 1 in, 2 out]
                    }
                    frame #1 {
                      n236 = Wait (ms)(milliseconds to wait="DAQ Delay (ms)") -> ()  [unwired: 1 out]
                    }
                    frame #2 {
                      n237 = local read "Slow mean"() -> (w442:dbl)
                      n238 = local read "Sigma"() -> (w441:dbl)
                    }
                  }
                }
                n239 = Bundle("Begin (V)"="Begin (V)", w408, w414) -> (→"MCL Scan":cluster{"Begin (V)":dbl, dbl, dbl[]})  [unwired: 1 out]
                n240 = Bundle("Begin (V)"="Begin (V)", w408, w407) -> (→"MCL Scan 2":cluster{"Begin (V)":dbl, dbl, dbl[]})  [unwired: 1 out]
              }
            }
          }
        }
        n241 = local read "Stop All"() -> (w352:bool)
        n242 = node-c288() -> ()  [unwired: 2 out]
      }
      n243 = node-c288(w349) -> ()  [unwired: 1 out]
    }
    frame Enabled {
    }
  }
  n244 = node-c288(3 ("Processor")) -> (w106:T21)  [unwired: 3 out]
  n245 = timed-loop "Oscillate Trap/AOM (fishing, debugging)" {
    tunnel: w18 -> [w446]
    tunnel: [w445] -> w111
    timing: w106 -> [_]
    timing-out: [_] -> w105
    stop <- w445 stop-if-true
    n246 = node-c288() -> ()  [unwired: 2 out]
    n247 = event shown="[1] \"Fl. Triggered...\": Value Change" {
      selector: _ -> [_ _ _]
      dyn-events: _ -> [_ _ _]
      timeout: _ -> [_ _ _]
      tunnel: w446 -> [w453 _ _]
      tunnel: [FALSE ("Stop All") _ w1134] -> w445
      event "Oscillate Set 1", "Fish": Value Change {
        n248 = event-data() -> ()  [unwired: 6 out]
        n249 = local read "Oscillate Set 1"() -> (w452:bool)
        n250 = Or(x=w452, y="Fish") -> (x .or. y?=w450:bool)
        n251 = case shown="True" w450 {
          tunnel: w453 -> [_ w456]
          tunnel: "Fish" -> [_ w454]
          frame False {
          }
          frame True {
            n252 = case shown="True" w454 {
              selector: w454 -> [w459 w460]
              tunnel: [w459 w460] -> w455
              frame False {
              }
              frame True {
                w461 = FALSE ("Tether")
                n253 = local write "Scan axis 2"(TRUE) -> ()
                n254 = local write "Tether"(w461) -> ()
                n255 = local write "Hysteresis"(w461) -> ()
                n256 = local write "Multiple tether"(w461) -> ()
                n257 = local write "Bad fit"(w461) -> ()
                n258 = local write "Good tether"(w461) -> ()
                n259 = property on="Trap D (MHz)" class="DigNum (strict)"("Val(Sgnl)"="Furthest D (MHz)") -> ()  [unwired: 2 in, 2 out]
                n260 = local read "Flow ON\nduring cal?"() -> (w462:bool)
                n261 = Or(x="Flow ON during \nfishing?", y=w462) -> (x .or. y?=w463:bool)
                n262 = Wait (ms)(milliseconds to wait=u32 500) -> ()  [unwired: 1 out]
                n263 = property on="Sample Channel\nFlow" class="Bool (strict)"("Val(Sgnl)"=w463) -> ()  [unwired: 2 in, 2 out]
              }
            }
            n264 = node-c288() -> (w458:T21)  [unwired: 4 out]
            n265 = timed-loop "Oscillate AOD" {
              timing: w458 -> [_]
              timing-out: [_] -> w457
              tunnel: w456 -> [w475]
              tunnel: w455 -> [w469]
              i -> [w477]
              stop <- w468 stop-if-true
              n266 = node-c288() -> (w476:i64)  [unwired: 1 out]
              n267 = flat-sequence {
                tunnel: w477 -> [w504]
                tunnel: w476 -> [w503]
                tunnel: w475 -> [w482]
                tunnel: w469 -> [w485]
                tunnel: [w485] -> w474
                tunnel: [w484] -> w473
                tunnel: [w481] -> w472
                tunnel: [w478] -> w470
                tunnel: w474 -> [w547]
                tunnel: w473 -> [w545]
                tunnel: w472 -> [w544]
                tunnel: [w543] -> w471
                tunnel: w470 -> [w542]
                tunnel: [w699] -> w468
                tunnel: w471 -> [w698]
                frame #0 {
                  n268 = Divide(x=w503, y=i64 1000) -> (x/y=w498:dbl)
                  n269 = Multiply(x=w498, y=w504) -> (x*y=w500:dbl)
                  n270 = local read "BD 1 Frequency 2 (MHz)"() -> (w483:dbl)
                  n271 = Multiply(x="Osc. freq. (Hz)", y=6.283185307179586) -> (x*y=w501:dbl)
                  n272 = Multiply(x=w501, y=w500) -> (x*y=w480:dbl)
                  n273 = local read "BD 1 Frequency 1 (MHz)"() -> (w488:dbl)
                  n274 = local read "BD 2 Frequency 1 (MHz)"() -> (w487:dbl)
                  n275 = case shown="True" w485 {
                    tunnel: w480 -> [w510 w515]
                    tunnel: w488 -> [_ w526]
                    tunnel: w483 -> [_ w527]
                    tunnel: [w507 w521] -> w486
                    tunnel: [FALSE w518] -> w481
                    tunnel: [0.0 w511] -> w478
                    frame False {
                      n276 = Sine(x=w510) -> (sin(x)=w508:dbl)
                      n277 = Multiply(x=w508, y="Osc. amp. (MHz)") -> (x*y=w507:dbl)
                    }
                    frame True {
                      n278 = Cosine(x=w515) -> (cos(x)=w530:dbl)
                      n279 = Subtract(x=w527, y=w526) -> (x-y=w525:dbl)
                      n280 = Decrement(x=w530) -> (x-1=w529:dbl)
                      n281 = Subtract(x=w525, y="Closest D (MHz)") -> (x-y=w522:dbl)
                      n282 = Divide(x=w529, y=-2.0) -> (x/y=w523:dbl)
                      n283 = Multiply(x=w523, y=w522) -> (x*y=w521:dbl)
                      n284 = local read "Vec Mean of T1 T2"() -> (w517:dbl[])
                      n285 = Greater?(x=w517, y="Stop F (pN)") -> (0:w519:bool[])
                      n286 = Or Array Elements(Boolean array=w519) -> (logical OR=w518:bool)
                      n287 = Divide(x=w515, y=6.283185307179586) -> (x/y=w514:dbl)
                      n288 = Round Toward +Infinity(x=w514) -> (ceil(x): smallest int >= x=w511:dbl)
                      "Attempts" <- w511
                      n289 = Greater?(x=w511, y="Attempt Limit") -> (0:w513:bool)
                      n290 = case shown="True" w513 {
                        frame False {
                        }
                        frame True {
                          n291 = local write "Fish"(FALSE ("Fish for Tether")) -> ()
                          n292 = local read "Messages"() -> (w532:string)
                          n293 = flat-sequence {
                            frame #0 {
                              n294 = call <vilib>:"Beep.vi"("use system alert? (T)"=FALSE, "duration (msec)"=u32 200, "frequency (Hz)"=u32 500) -> ()  [unwired: 9 out]
                            }
                            frame #1 {
                              n295 = Wait (ms)(milliseconds to wait=u32 100) -> ()  [unwired: 1 out]
                            }
                            frame #2 {
                              n296 = call <vilib>:"Beep.vi"("use system alert? (T)"=FALSE, "duration (msec)"=u32 200, "frequency (Hz)"=u32 500) -> ()  [unwired: 9 in]
                            }
                          }
                          n297 = call "Update messages.vi"("Message to add"="Tether fishing timeout." ("Messages"), "Old message string"=w532) -> ("New message string"=→"Messages":string)
                        }
                      }
                    }
                  }
                  n298 = Select(t=w488, s="Scan axis 2", f=w487) -> (s? t:f=w491:dbl)
                  n299 = Add(x=w486, y=w491) -> (x+y=w484:dbl)
                  n300 = Select(t=w484, s="Scan axis 2", f=w488) -> (s? t:f=w494:dbl)
                  n301 = Select(t=w487, s="Scan axis 2", f=w484) -> (s? t:f=w493:dbl)
                  n302 = local read "Y RF Frequency Limits (MHz)"() -> (w489:T16)
                  n303 = local read "X RF Frequency Limits (MHz)"() -> (w490:T16)
                  n304 = local read "BD 2 Frequency 2 (MHz)"() -> (w496:dbl)
                  n305 = local read "BD 2 Frequency 3 (MHz)"() -> (w495:dbl)
                  n306 = local read "BD 1 Frequency 3 (MHz)"() -> (w497:dbl)
                  n307 = call "set RF board frequency - interlace.vi"("Board 2 Frequency Limits"=w489, "Board 1 Frequency Limits"=w490, "FPGA VI Reference In"=w482, "Board 2 Frequency 3 (MHz)"=w495, "Board 1 Frequency 3 (MHz)"=w497, "Board 2 Frequency 2 (MHz)"=w496, "Board 2 Frequency 1 (MHz)"=w493, "Board 1 Frequency 2 (MHz)"=w483, "Board 1 Frequency 1  (MHz)"=w494) -> ()  [unwired: 1 in, 2 out]
                }
                frame #1 {
                  n308 = And(x=w547, y=w544) -> (x .and. y?=w546:bool)
                  n309 = case "Only if were fishing and now formed tether" shown="True" w546 {
